vi "Image To String.vi"(7 "错误输入（无错误）":errorcluster, 10 "引用句柄输入":T1) -> (0 "错误输出":errorcluster, 1 "FileString":string, 3 "引用句柄输出":T1)   [LabVIEW 2017, in "Encode Base64.lvlib"]
uses:
  Encode Base64.lvlib
  <vilib>/vision/NI_Vision_Development_Module.lvlib
  <vilib>/vision/Image Controls.llb/IMAQ Image.ctl
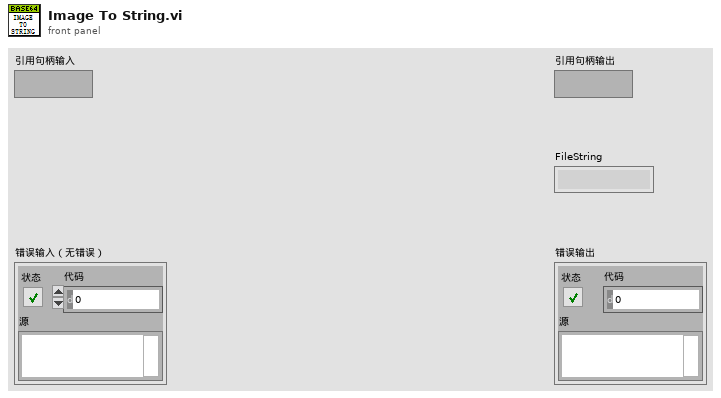
[diagram p1: front panel]
types:
  T1 = typedef "IMAQ Image.ctl" = refnum<image>
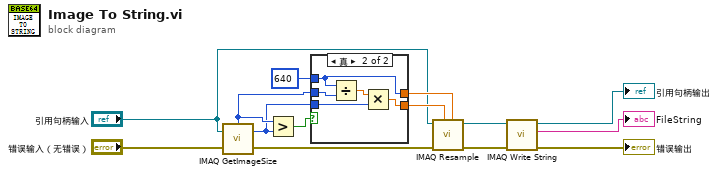
[diagram p0: block diagram]
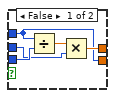
[diagram p2: hidden frame]
diagram:
  n1 = call "IMAQ GetImageSize"("Image"="引用句柄输入", "error in (no error)"="错误输入（无错误）") -> ("Y Resolution"=w5:i32, "X Resolution"=w6:i32, "error out"=w9:errorcluster)  [unwired: 2 in]
  n2 = Greater?(x=w6, y=w5) -> (0:w7:bool)
  n3 = case shown="真" w7 {
    tunnel: w6 -> [w17 w24]
    tunnel: w5 -> [w19 w23]
    tunnel: [w15 w21] -> w4
    tunnel: 640 ("x") -> [w15 w20]
    tunnel: [w16 w20] -> w2
    frame False {
      n4 = Divide(x=w15, y=w19) -> (x/y=w18:dbl)
      n5 = Multiply(x=w18, y=w17) -> (x*y=w16:dbl)
    }
    frame True {
      n6 = Divide(x=w20, y=w24) -> (x/y=w22:dbl)
      n7 = Multiply(x=w22, y=w23) -> (x*y=w21:dbl)
    }
  }
  n8 = call "IMAQ Resample"("X Resolution"=w2, "Y Resolution"=w4, "error in (no error)"=w9, "Image Src"="引用句柄输入") -> ("error out"=w8:errorcluster, "Image Dst Out"=w14:T1)  [unwired: 6 in]
  n9 = call-poly "IMAQ Write String"("error in (no error)"=w8, "Image"=w14) -> ("error out"=→"错误输出":errorcluster, "FileString"=→"FileString":string, "Image Out (duplicate)"=→"引用句柄输出":T1)  [unwired: 7 in]
